vi "in_order_traverse.vi"(7 "tree":refnum<vi>, 8 "error in (no error)":errorcluster, 10 "node":string="L 22", 11 "all data":i32[](array[numeric])) -> (0 "error out":errorcluster, 3 "all data out":i32[](array[numeric]))   [LabVIEW 2021]
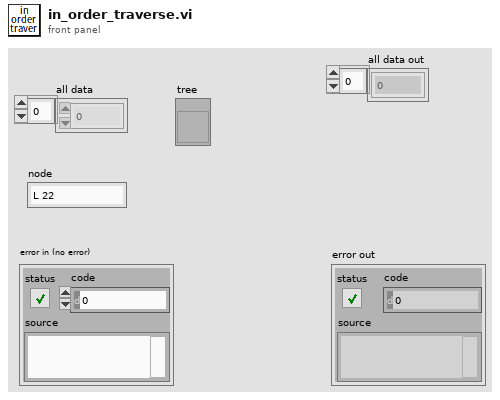
[diagram p1: front panel]
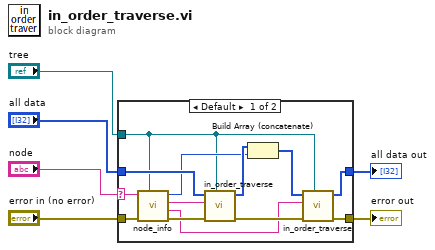
[diagram p0: block diagram]
diagram:
  n1 = case shown="Default" "node" {
    selector: "node" -> [w19 _]
    tunnel: "all data" -> [w16 w21]
    tunnel: [w8 w21] -> w5
    tunnel: "tree" -> [w11 _]
    tunnel: "error in (no error)" -> [w18 w20]
    tunnel: [w7 w20] -> w1
    frame Default {
      n2 = call "node_info.vi"("reference"=w11, "error in (no error)"=w18, "node"=w19) -> ("error out"=w17:errorcluster, "right"=w9:string, "left"=w15:string, "value"=w13:i32)  [unwired: 5 in]
      n3 = call "in_order_traverse.vi"("tree"=w11, "error in (no error)"=w17, "node"=w15, "all data"=w16) -> ("error out"=w10:errorcluster, "all data out"=w14:i32[])  [unwired: 6 in]
      n4 = Build Array (concatenate)(w14, w13) -> (w12:i32[])
      n5 = call "in_order_traverse.vi"("tree"=w11, "error in (no error)"=w10, "node"=w9, "all data"=w12) -> ("error out"=w7:errorcluster, "all data out"=w8:i32[])  [unwired: 6 in]
    }
    frame "" {
    }
  }
  "all data out" <- w5
  "error out" <- w1
